vi "_RDB_VI_Tree.vi"   [LabVIEW 2023, in "RDB.lvlib"]
uses:
  RDB.lvlib
  Shared/Compiled.Settings.ctl
  System Explorer/RDB Data.ctl
  RDB Object.ctl
  RDB Player Object.ctl
  Shared/Network Settings.ctl
  Shared/Protocol.ctl
  Shared/SensorInfos.ctl
  Shared/SensorInfo.ctl
  Shared/Sensor Name.ctl
  MM/MM Data.ctl
  MM/MM Objects.ctl
  MM/MM Object.ctl
  Shared/Timedloop Settings.ctl
  Shared/Vires VTD Shared.lvlib
  MM/MM.lvlib
types:
  T1 = typedef "Vires VTD Shared.lvlib/Compiled.Settings.ctl" = cluster{"Name":string, "RDB Data Receive ":T2, "RDB Data Sent":T2, "vclient":path, "Network Settings":T5, "SensorInfos":T7, "mmanager":path, "Scenario Paths":string[], "Custom SCP Commands":string[], "Timed Loop Settings for TaskControl":T13, "Timed Loop Settings for ModuleManager":T13}
  T2 = typedef "Vires VTD Shared.lvlib/RDB Data.ctl" = T3[]
  T3 = typedef "RDB.lvlib/RDB Object.ctl" = cluster{"pkID":i32, "RDB Player Objects":T4[]}
  T4 = typedef "RDB.lvlib/RDB Player Object.ctl" = cluster{"PlayerID":i32, "Signals":string[], "adv para":i32}
  T5 = typedef "Vires VTD Shared.lvlib/Network Settings.ctl" = cluster{"IP adress":string, "RDB":cluster{"Protocol":T6, "Tx Port":u16, "Rx Port":u16, "Buffer Size":i32, "Timeout":u16}, "SCP":cluster{"Protocol":T6, "Tx Port":u16, "Rx Port":u16, "Buffer Size":i32, "Timeout":u16}}
  T6 = typedef "Vires VTD Shared.lvlib/Protocol.ctl" = enum16{"UDP", "TCP"}
  T7 = typedef "Vires VTD Shared.lvlib/SensorInfos.ctl" = T8[]
  T8 = typedef "Vires VTD Shared.lvlib/SensorInfo.ctl" = cluster{"Sensor Name":T9, "Protocol":T6, "Network port":i32, "# Culled Objects":i32, "PlayerID":u8, "MM Data":T10}
  T9 = typedef "Vires VTD Shared.lvlib/Sensor Name.ctl" = string
  T10 = typedef "Vires VTD Shared.lvlib/MM Data.ctl" = T11[]
  T11 = typedef "MM.lvlib/MM Objects.ctl" = cluster{"pkID":i32, "MM Objects":T12[]}
  T12 = typedef "MM.lvlib/MM Object.ctl" = cluster{"Object":i32, "Signals":string[]}
  T13 = typedef "Vires VTD Shared.lvlib/Timedloop Settings.ctl" = cluster{"Period(ms)":i64, "Priority":i32, "Processor":i32}
  T14 = typedef "Vires VTD Engine.lvlib/Settings.ctl" = cluster{"UDP Receiver":refnum<k16>, "UDP Sender":refnum<k16>, "Valid Packet":bool, "TCP":refnum<k5>, "Network Settings":T5, "vclient":path, "paeseHandle":u64, "builderHandle":u64}
  T15 = typedef "RDB.lvlib/RDB References.ctl" = cluster{"RDB Receive Reference":T16, "RDB Send Reference":T16}
  T16 = typedef "RDB.lvlib/RDB Reference.ctl" = cluster{"Conversion References":refnum<k21>[], "RDB Data":T17[], "RDB Signals":dbl[], "noSignals":i32[]}
  T17 = typedef "XNET Frame FlexRay.ctl" = cluster{"timestamp":timestamp, "payload":u8[], "slot":u16, "type":T18, "cycle count":u8, "startup?":bool, "sync?":bool, "preamble?":bool, "ch A":bool, "ch B":bool, "echo?":bool}
  T18 = typedef "XNET Frame Type FlexRay.ctl" = u8
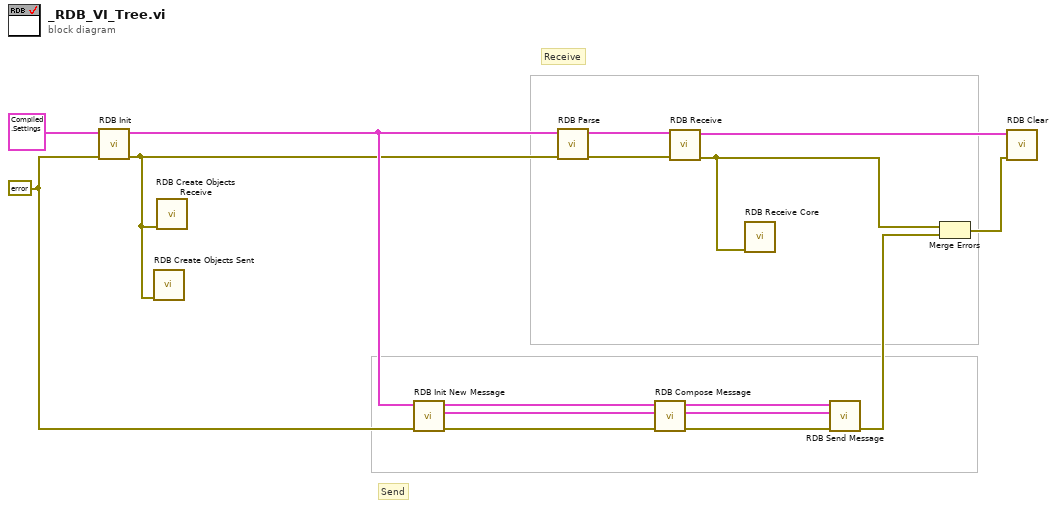
[diagram p0: block diagram]
diagram:
  w3 = errorcluster {"status"=FALSE, "code"=0, "source"=""} ("error in")
  # "Send"
  # "Receive"
  n1 = call "RDB Init.vi"("error in"=w3, "Compiled.Settings"=T1 {"Name"="", "RDB Data Receive "=[], "RDB Data Sent"=[], "vclient"=path "", "Network Settings"={"IP adress"="127.0.0.1", "RDB"={"Protocol"=enum."UDP", "Tx Port"=48270, "Rx Port"=10, "Buffer Size"=204800, "Timeout"=10}, "SCP"={"Protocol"=enum."TCP", "Tx Port"=48191, "Rx Port"=48191, "Buffer Size"=204800, "Timeout"=10}}, "SensorInfos"=[], "mmanager"=path "", "Scenario Paths"=[], "Custom SCP Commands"=[], "Timed Loop Settings for TaskControl"={"Period(ms)"=2, "Priority"=100, "Processor"=-2}, "Timed Loop Settings for ModuleManager"={"Period(ms)"=2, "Priority"=100, "Processor"=-2}}) -> ("error out"=w4:errorcluster, "Settings"=w14:T14)  [unwired: 7 in, 1 out]
  n2 = call "RDB Create Objects Sent.vi"("error in (no error)"=w4) -> ()  [unwired: 9 in, 2 out]
  n3 = call "RDB Create Objects Receive.vi"("error in (no error)"=w4) -> ()  [unwired: 9 in, 2 out]
  n4 = call "RDB Init New Message.vi"("error in (no error)"=w3, "Settings"=w14) -> ("error out"=w8:errorcluster, "RDB Reference out"=w1:T15, "Settings"=w10:T14)  [unwired: 7 in]
  n5 = call "RDB Parse.vi"("error in (no error)"=w4, "Settings"=w14) -> ("error out"=w13:errorcluster, "Settings"=w16:T14)  [unwired: 6 in, 2 out]
  n6 = call "RDB Compose Message.vi"("error in (no error)"=w8, "RDB Reference in"=w1, "Settings"=w10) -> ("error out"=w7:errorcluster, "RDB Reference out"=w2:T15, "Settings"=w9:T14)  [unwired: 6 in]
  n7 = call "RDB Receive.vi"("error in (no error)"=w13, "Settings"=w16) -> ("error out"=w5:errorcluster, "Settings"=w12:T14)  [unwired: 7 in, 1 out]
  n8 = call "RDB Receive Core.vi"("error in (no error)"=w5) -> ()  [unwired: 8 in, 3 out]
  n9 = call "RDB Send Message.vi"("error in (no error)"=w7, "RDB Reference in"=w2, "Settings"=w9) -> ("error out"=w6:errorcluster)  [unwired: 5 in, 3 out]
  n10 = Merge Errors(w5, w6) -> (w11:errorcluster)
  n11 = call "RDB Clear.vi"("error in (no error)"=w11, "Settings"=w12) -> ()  [unwired: 9 in, 1 out]
